vi "call service in ros.vi"(7 "error in (no error)":errorcluster, 10 "TCP Network Connection in":refnum<k5>) -> (0 "error out":errorcluster, 3 "TCP Network Connection out":refnum<k5>, 4 "founded STEERING":bool)   [LabVIEW 2015]
uses:
  <vilib>/MediaMongrels Ltd/WebSockets/WebSockets/WebSockets.lvlib
panel:
  out "ros call service return":T1
  in  "ros call service ctl.":T1
  out "Data":string
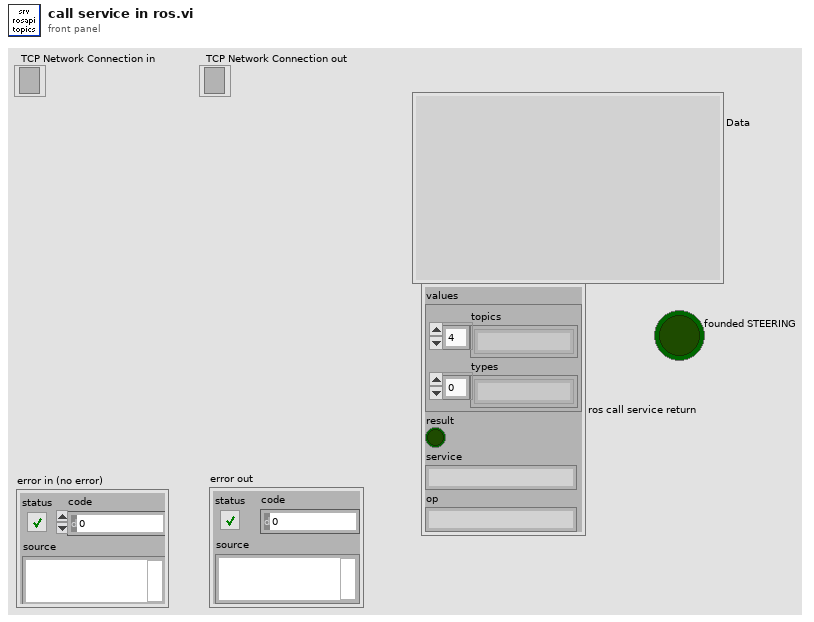
[diagram p1: front panel]
types:
  T1 = cluster{"values":cluster{"topics":string[], "types":string[]}, "result":bool, "service":string, "op":string}
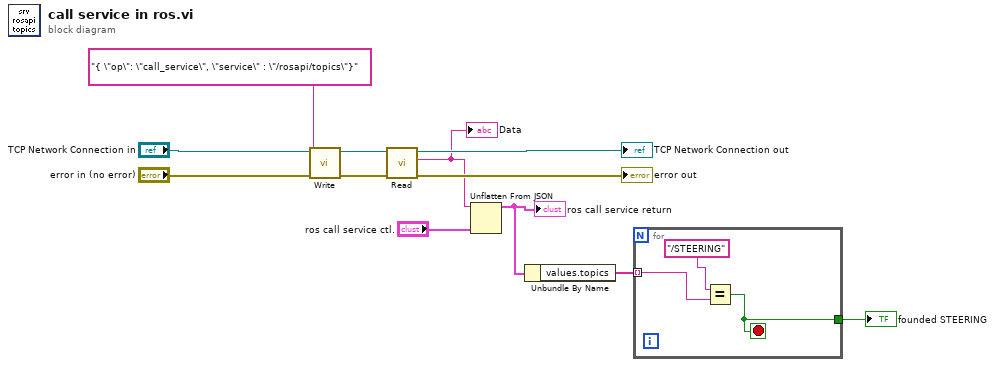
[diagram p0: block diagram]
diagram:
  n1 = call <vilib>:"Write.vi"("error in (no error)"="error in (no error)", "Data"="{ \"op\": \"call_service\", \"service\" : \"/rosapi/topics\"}", "WebSocket Connection in"="TCP Network Connection in") -> ("error out"=w9:errorcluster, "WebSocket Connection out"=w8:refnum<k5>)  [unwired: 7 in]
  n2 = call <vilib>:"Read.vi"("error in (no error)"=w9, "WebSocket Connection in"=w8) -> ("error out"=→"error out":errorcluster, "Data"=w5:string, "WebSocket Connection out"=→"TCP Network Connection out":refnum<k5>)  [unwired: 6 in, 1 out]
  "Data" <- w5
  n3 = Unflatten From JSON(JSON string=w5, type and defaults="ros call service ctl.") -> (value=w3:T1)  [unwired: 5 in, 1 out]
  "ros call service return" <- w3
  n4 = Unbundle By Name(w3) -> ("values.topics"=w2:string[])
  n5 = for {
    tunnel: w2 -> [w15] mode=indexing
    tunnel: [w13] -> w1
    stop <- w13 stop-if-true
    n6 = Equal?(x="/STEERING", y=w15) -> (x = y?=w13:bool)
  }
  "founded STEERING" <- w1
